vi "Release-message-queues.vi"(8 "error in (no error)":errorcluster, 11 "Object ref in":T1) -> (0 "error out":errorcluster, 3 "Object ref out":T1)   [LabVIEW 2013, in "HardwareCharacterization.lvlib" / "HC-Main.lvclass"]
uses:
  HC-Main.lvclass
  Object-reference.ctl
  HC-Main.lvclass/HC-Main.ctl
  Read Action queue.vi
  Read Process 1 queue.vi
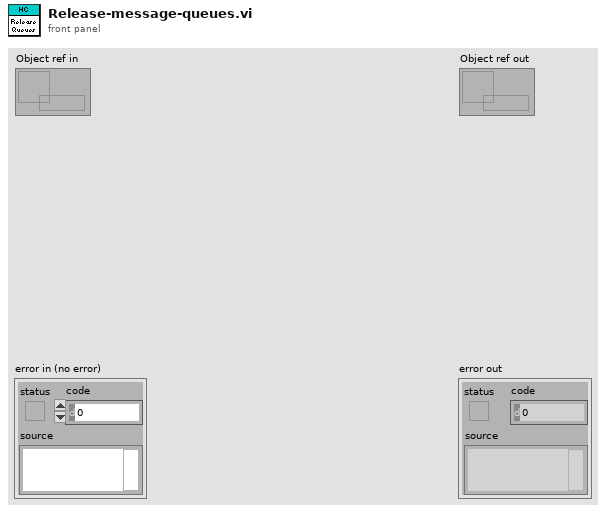
[diagram p1: front panel]
types:
  T1 = typedef "HardwareCharacterization.lvlib/HC-Main.lvclass/Object-reference.ctl" = refnum<data-value>
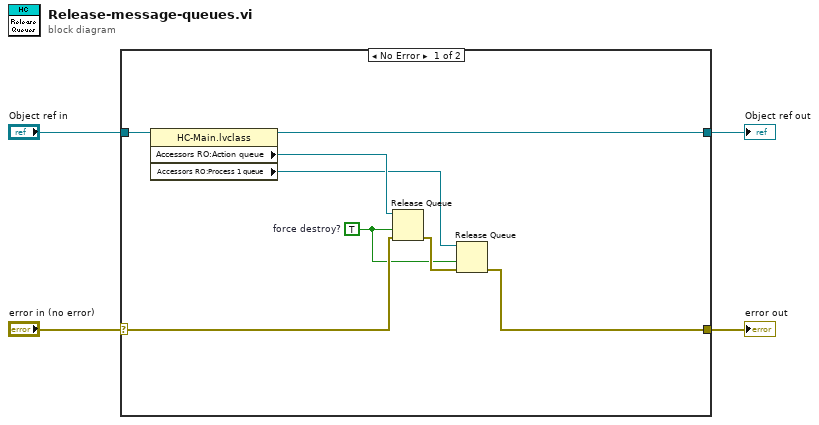
[diagram p0: block diagram]
diagram:
  n1 = case shown="No Error" "error in (no error)" {
    selector: "error in (no error)" -> [w9 w14]
    tunnel: [w5 w14] -> w3
    tunnel: [w11 w13] -> w1
    tunnel: "Object ref in" -> [w12 w13]
    frame No Error {
      w6 = TRUE  # force destroy?
      n2 = property class="HC-Main.lvclass"(reference=w12) -> (reference out=w11:T1, "Accessors RO:Action queue"=w10:refnum<queue>, "Accessors RO:Process 1 queue"=w8:refnum<queue>)  [unwired: 1 in, 1 out]
      n3 = Release Queue(queue=w10, force destroy? (F)=w6, error in (no error)=w9) -> (error out=w7:errorcluster)  [unwired: 2 out]
      n4 = Release Queue(queue=w8, force destroy? (F)=w6, error in (no error)=w7) -> (error out=w5:errorcluster)  [unwired: 2 out]
    }
    frame Error {
    }
  }
  "error out" <- w3
  "Object ref out" <- w1
